vi "check saved scan files.vi"() -> ()   [LabVIEW 2020]
panel:
  out "All equal":bool caption="All diags same # shots"
  out "folder info":cluster{string, i32}[](array[cluster])
  in  "scan path":path
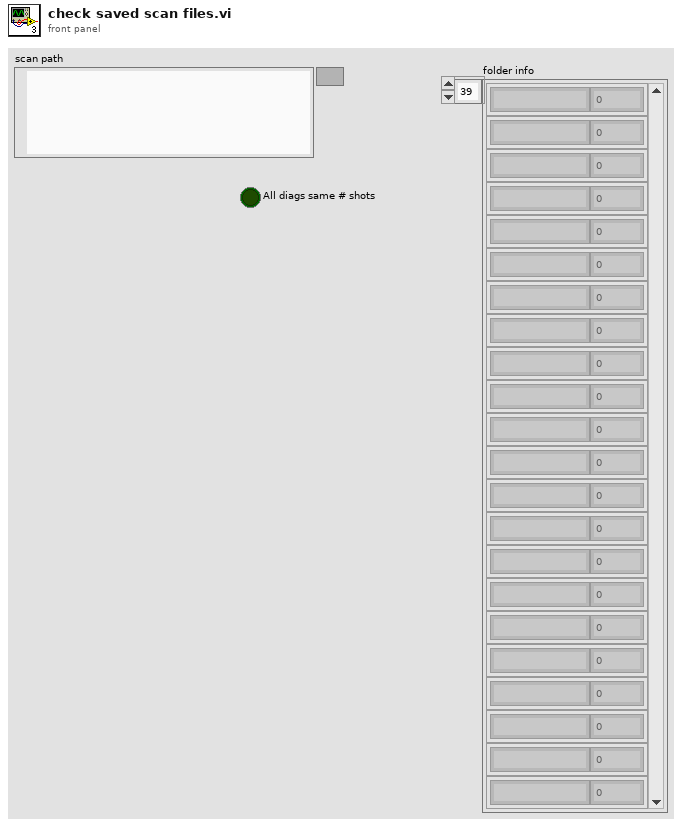
[diagram p1: front panel]
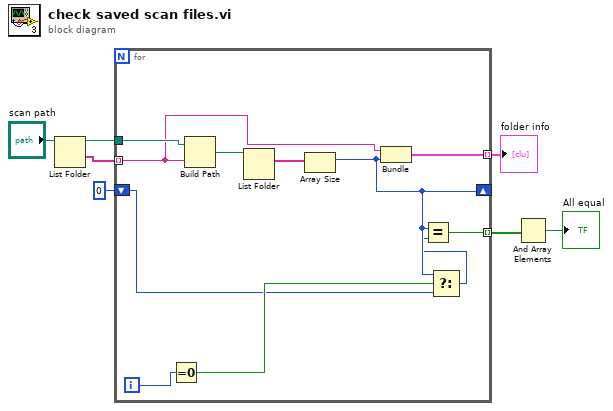
[diagram p0: block diagram]
diagram:
  n1 = List Folder(path="scan path") -> (path out=w5:path, folder names=w6:string[])  [unwired: 3 in, 2 out]
  n2 = for {
    tunnel: w6 -> [w15] mode=indexing
    tunnel: w5 -> [w18]
    tunnel: [w14] -> w4 mode=indexing
    shift-right: [w11] -> _
    shift-left: 0 -> [w10]
    tunnel: [w8] -> w2 mode=indexing
    i -> [w13]
    n3 = Equal To 0?(x=w13) -> (x = 0?=w12:bool)
    n4 = Build Path(base path=w18, name or relative path=w15) -> (appended path=w17:path)
    n5 = List Folder(path=w17) -> (filenames=w16:string[])  [unwired: 3 in, 3 out]
    n6 = Array Size(array=w16) -> (size(s)=w11:i32)
    n7 = Bundle(w15, w11) -> (w14:cluster{string, i32})  [unwired: 1 in]
    n8 = Select(t=w11, s=w12, f=w10) -> (s? t:f=w9:i32)
    n9 = Equal?(x=w11, y=w9) -> (x = y?=w8:bool)
  }
  "folder info" <- w4
  n10 = And Array Elements(Boolean array=w2) -> (logical AND=→"All equal":bool)
